vi "Log Error.vi"(8 "error in (no error)":errorcluster, 10 "Level":T1, 11 "Application Log in":refnum<class "Application Log.lvclass">) -> (0 "error out":errorcluster, 2 "Error Message":string, 3 "Application Log out":refnum<class "Application Log.lvclass">)   [LabVIEW 2016, in "Stream Log.lvlib" / "Application Log.lvclass"]
doc: "--\nCopyright © 2017 Composed SystemsI All rights reserved.\n\nAuthor: Jon McBee <jon.mcbee@composed.io>\n\nThis library is provided \"AS IS\" ,WITHOUT WARRANTIES OR\nCONDITIONS OF ANY KIND, either express or implied.\n\nComposed Systems -- composed.io\n\nStream 0.0.1.1\nJon McBee - Composed Systems\nCopyright (c) 2017, Composed Systems"
uses:
  <userlib>/Composed Systems/Stream/Log/Application Log/Application Log.lvclass
  <userlib>/Composed Systems/Stream/Log/Application Log/Log Level.ctl
  <userlib>/Composed Systems/Stream/Log/Application Log/Application Log.lvclass/Application Log.ctl
  <userlib>/Composed Systems/Stream/Error/Stream Error.lvlib
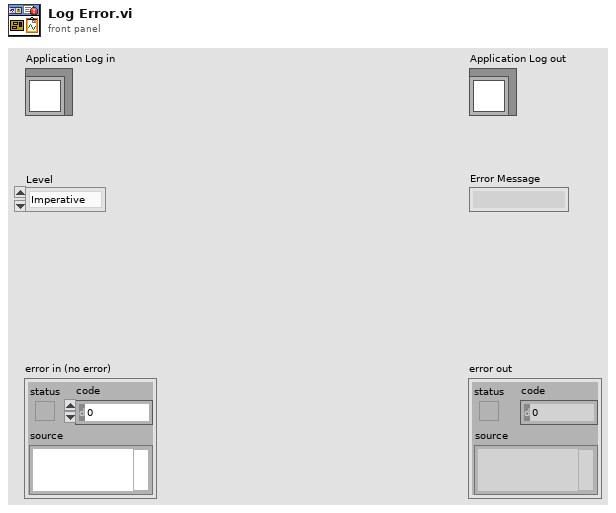
[diagram p1: front panel]
types:
  T1 = typedef "Stream Log.lvlib/Application Log.lvclass/Log Level.ctl" = enum16{"Imperative", "Major", "Minor", "Debug", "Off"}
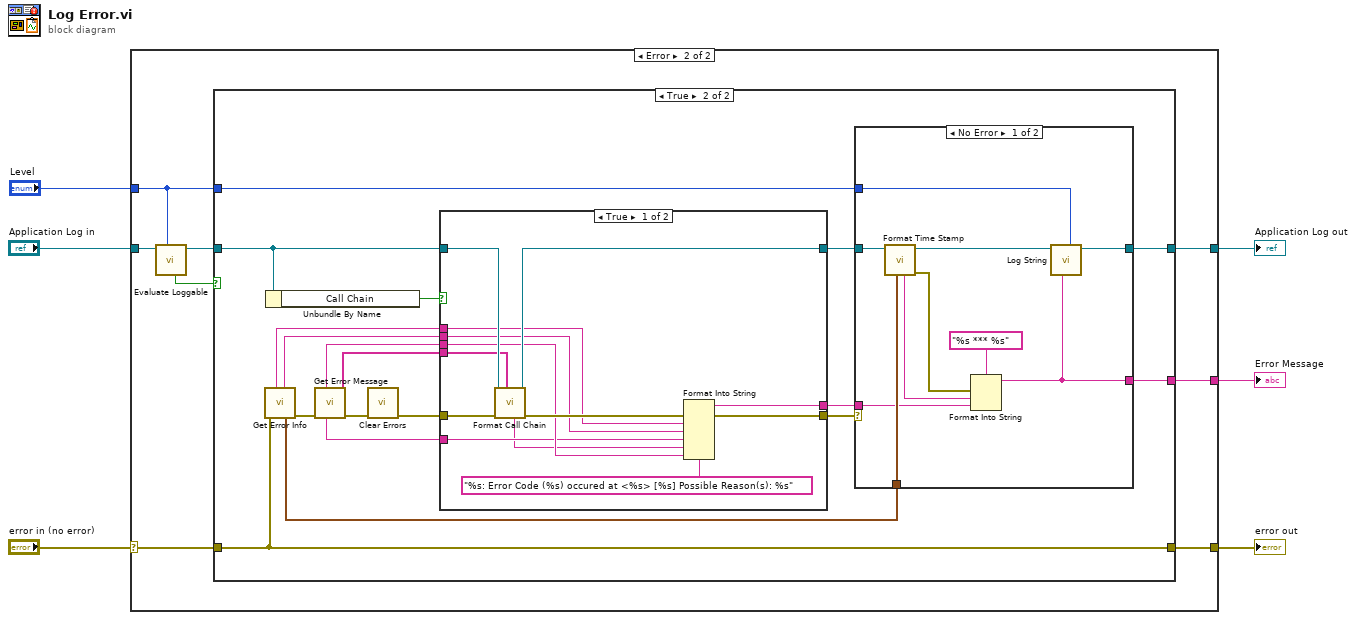
[diagram p0: block diagram]
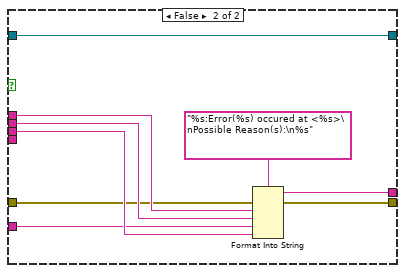
[diagram p5: hidden frame]
diagram:
  n1 = case shown="Error" "error in (no error)" {
    selector: "error in (no error)" -> [w8 w15]
    tunnel: [w8 w14] -> w5
    tunnel: [w7 w16] -> w3
    tunnel: "Application Log in" -> [w7 w13]
    tunnel: "Level" -> [_ w10]
    tunnel: [_ w9] -> w1
    frame No Error {
    }
    frame Error {
      n2 = call <userlib>:"Evaluate Loggable.vi"("Level"=w10, "Application Log in"=w13) -> ("Application Log out"=w12:refnum<class "Application Log.lvclass">, "Log?"=w11:bool)  [unwired: 8 in]
      n3 = case shown="True" w11 {
        tunnel: [w18 w33] -> w16
        tunnel: w12 -> [w18 w35]
        tunnel: [w17 w25] -> w14
        tunnel: w15 -> [w17 w25]
        tunnel: w10 -> [_ w30]
        tunnel: [_ w29] -> w9
        frame False {
        }
        frame True {
          n4 = call <userlib>:"Get Error Info.vi"("Error In"=w25) -> ("Error Out"=w24:errorcluster, "Time Stamp"=w26:timestamp, "Error Name"=w27:string, "Error Scope"=w28:string)  [unwired: 6 in, 1 out]
          n5 = Unbundle By Name(w35) -> ("Call Chain"=w36:bool)
          n6 = call <userlib>:"Get Error Message.vi"("Error In"=w24) -> ("Error Out"=w23:errorcluster, "Call Chain"=w20:string[], "Error Source"=w21:string, "Error Message"=w22:string)  [unwired: 6 in, 1 out]
          n7 = call <vilib>:"Clear Errors.vi"("error in (no error)"=w23) -> ("error out"=w19:errorcluster)  [unwired: 5 in, 1 out]
          n8 = case shown="True" w36 {
            tunnel: [w58 w62] -> w34
            tunnel: w35 -> [w59 w62]
            tunnel: w19 -> [w60 w61]
            tunnel: w28 -> [w53 w67]
            tunnel: w27 -> [w52 w66]
            tunnel: w22 -> [w51 w65]
            tunnel: w20 -> [w57 _]
            tunnel: w21 -> [w50 w64]
            tunnel: [w55 w69] -> w32
            tunnel: [w48 w63] -> w31
            frame True {
              n9 = call <userlib>:"Format Call Chain.vi"("Call Chain"=w57, "error in (no error)"=w60, "Application Log in"=w59) -> ("error out"=w56:errorcluster, "Application Log out"=w58:refnum<class "Application Log.lvclass">, "Formatted Call Chain"=w49:string)  [unwired: 6 in]
              n10 = Format Into String(format string="%s: Error Code (%s) occured at <%s> [%s] Possible Reason(s): %s", error in=w56, w53, w52, w50, w49, w51) -> (resulting string=w48:string, error out=w55:errorcluster)  [unwired: 1 in]
            }
            frame False {
              n11 = Format Into String(format string="%s:Error(%s) occured at <%s>\nPossible Reason(s):\n%s", error in=w61, w67, w66, w64, w65) -> (resulting string=w63:string, error out=w69:errorcluster)  [unwired: 1 in]
            }
          }
          n12 = case shown="No Error" w32 {
            tunnel: [w39 w47] -> w33
            tunnel: w34 -> [w46 w47]
            tunnel: w31 -> [w42 _]
            tunnel: w26 -> [w45 _]
            tunnel: w30 -> [w38 _]
            tunnel: [w37 _] -> w29
            frame No Error {
              n13 = call <userlib>:"Format Time Stamp.vi"("Time Stamp"=w45, "Application Log in"=w46) -> ("error out"=w41:errorcluster, "Application Log out"=w40:refnum<class "Application Log.lvclass">, "Formatted Time Stamp"=w43:string)  [unwired: 7 in]
              n14 = Format Into String(format string="%s *** %s", error in=w41, w43, w42) -> (resulting string=w37:string)  [unwired: 1 in, 1 out]
              n15 = call-dynamic "Log String.vi"("Level"=w38, "String"=w37, "Application Log in"=w40) -> ("Application Log out"=w39:refnum<class "Application Log.lvclass">)  [unwired: 7 in, 1 out]
            }
            frame Error {
            }
          }
        }
      }
    }
  }
  "error out" <- w5
  "Application Log out" <- w3
  "Error Message" <- w1
